vi "Source Step Delete.vi"(8 "error in (no error)":errorcluster, 10 "Step":T1=1 min=1 max=99 step=1, 11 "VISA resource name":refnum<visa-resource-name>) -> (0 "error out":errorcluster, 3 "VISA resource name out":refnum<visa-resource-name>)   [LabVIEW 2025, in "Chroma 19052.lvlib"]
doc: "Chroma\n5 Clock Tower Place Suite 210\nMaynard, MA 01754\nTel: 1 800 253-1230\nTel: 1 877 4 A HIPOT\nFax: 1 978-461-4295\nWebsite: www.chroma.com"
uses:
  <instrlib>/Chroma 19052/Chroma 19052.lvlib
  <instrlib>/Chroma 19052/Public/Utility/Type Def/steps--numeric.ctl
panel:
  # "Step Delete"
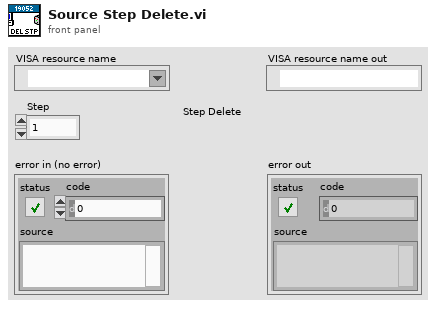
[diagram p1: front panel]
types:
  T1 = typedef "Chroma 19052.lvlib/steps--numeric.ctl" = u8
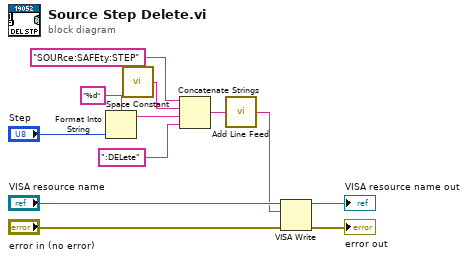
[diagram p0: block diagram]
diagram:
  n1 = Format Into String(format string="%d", "Step") -> (resulting string=w4:string)  [unwired: 2 in, 1 out]
  n2 = call <vilib>:"Space Constant.vi"() -> ("String"=w5:string)
  n3 = Concatenate Strings("SOURce:SAFEty:STEP", w5, w4, ":DELete") -> (w3:string)
  n4 = call <instrlib>:"Add Line Feed.vi"("Command string"=w3) -> ("Concatenated string"=w8:string)  [unwired: 4 in]
  n5 = VISA Write(VISA resource name="VISA resource name", write buffer=w8, error in (no error)="error in (no error)") -> (VISA resource name out=→"VISA resource name out":refnum<visa-resource-name>, error out=→"error out":errorcluster)  [unwired: 1 out]
